vi "LDA1_Safety.vi"(1 "Adam Loop Count":i32, 2 "Ch Names":string[](array[string]), 3 "Values":dbl[](array[numeric]) format="%.2f") -> (0 "Scan comment":string)   [LabVIEW 2014]
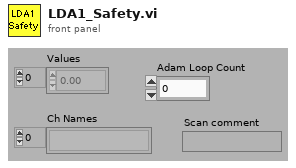
[diagram p1: front panel]
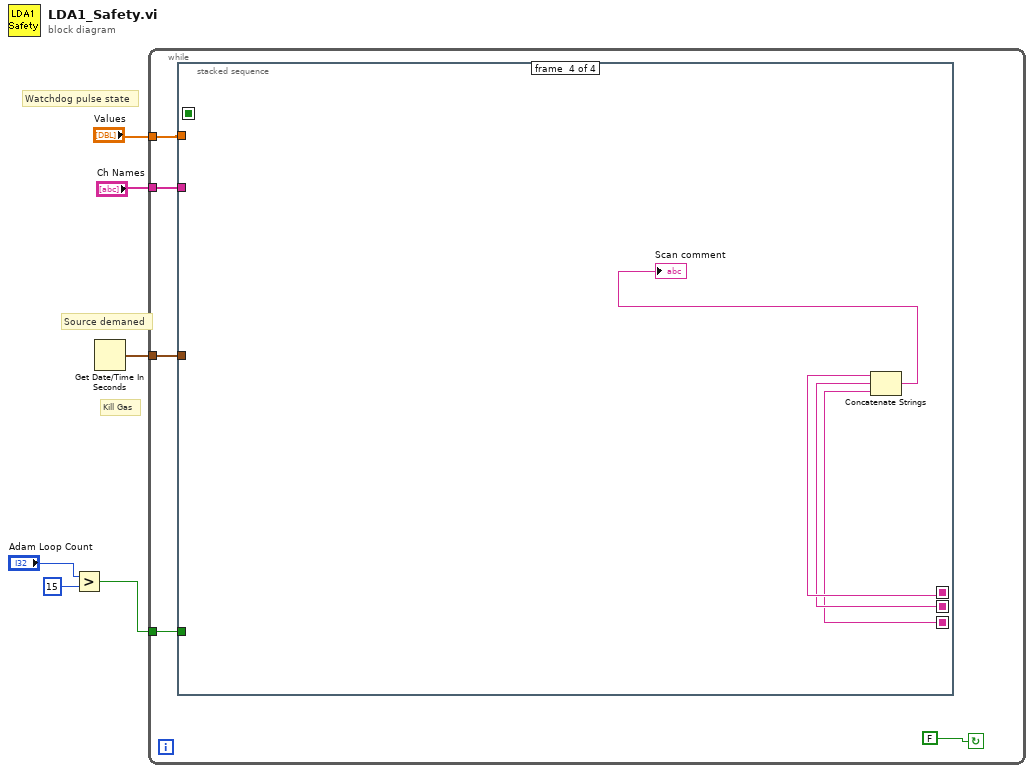
[diagram p0: block diagram]
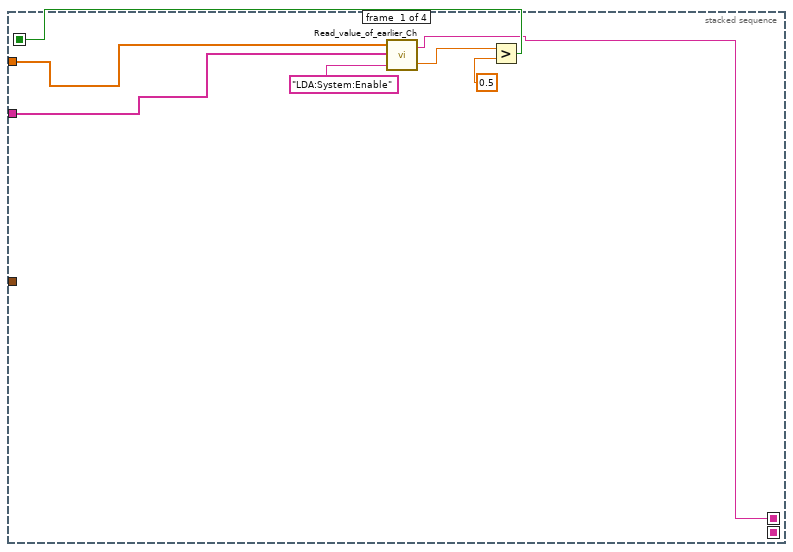
[diagram p2: hidden frame]
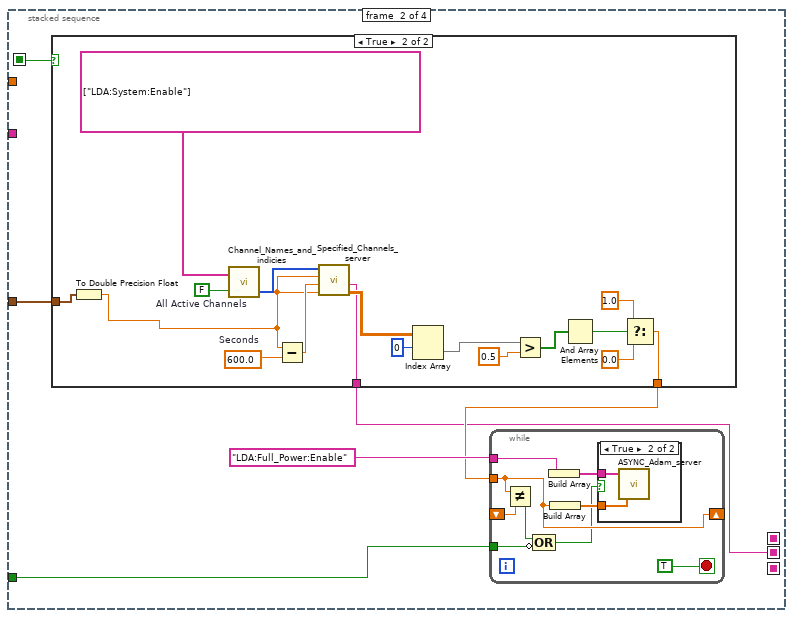
[diagram p3: hidden frame]
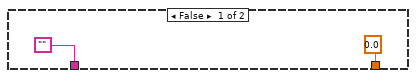
[diagram p5: hidden frame]
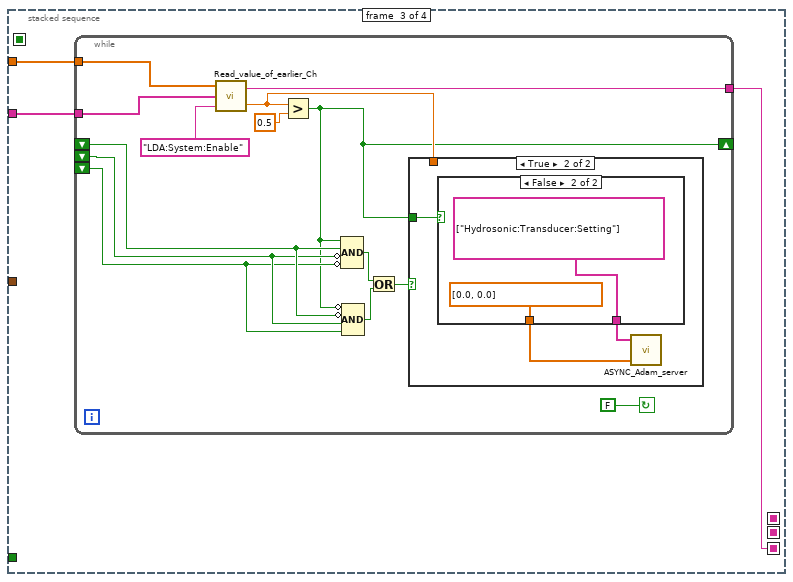
[diagram p6: hidden frame]
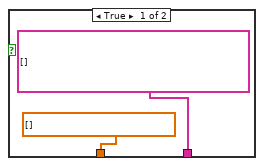
[diagram p8: hidden frame]
diagram:
  # "Source demaned"
  # "Watchdog pulse state"
  # "Kill Gas"
  n1 = Greater?(x="Adam Loop Count", y=15) -> (0:w2:bool)
  n2 = Get Date/Time In Seconds() -> (seconds since 1Jan1904=w1:timestamp)
  n3 = while {
    tunnel: "Ch Names" -> [w11]
    tunnel: "Values" -> [w10]
    tunnel: w2 -> [w8]
    tunnel: w1 -> [w7]
    stop <- FALSE continue-if-true
    n4 = stacked-sequence {
      seq-local: [w16 _ _ _] -> [_ w23 _ _]
      seq-local: [w12 _ _ _] -> [_ _ _ w82]
      seq-local: [_ w19 _ _] -> [_ _ _ w81]
      seq-local: [_ _ w55 _] -> [_ _ _ w80]
      tunnel: w11 -> [w17 _ w56 _]
      tunnel: w10 -> [w18 _ w57 _]
      tunnel: w8 -> [_ w21 _ _]
      tunnel: w7 -> [_ w24 _ _]
      frame #0 {
        n5 = call "Read_value_of_earlier_Ch.vi"("Desired Ch to Read"="LDA:System:Enable", "Ch names"=w17, "Present scan array"=w18) -> ("Value"=w14:dbl, "Scan comment"=w12:string)  [unwired: 1 in]
        n6 = Greater?(x=w14, y=0.5) -> (0:w16:bool)
      }
      frame #1 {
        n7 = case shown="True" w23 {
          tunnel: w24 -> [_ w54]
          tunnel: [0.0 ("y") w42] -> w20
          tunnel: ["" w39] -> w19
          frame False {
          }
          frame True {
            w52 = 600.0  # Seconds
            w50 = FALSE  # All Active Channels
            n8 = To Double Precision Float(number=w54) -> (double precision float=w48:dbl)
            n9 = call "Channel_Names_and_indicies.vi"("All Active Channels"=w50, "Desired Ch Names"=string[] ["LDA:System:Enable"]) -> ("Indicies"=w51:i32[])  [unwired: 1 out]
            n10 = Subtract(x=w48, y=w52) -> (x-y=w53:dbl)
            n11 = call "Specified_Channels_server.vi"("End time"=w48, "Start time"=w53, "Clients time"=w48, "Requested channels"=w51) -> ("Output array"=w46:dbl[][], "Messages"=w39:string)  [unwired: 1 in, 3 out]
            n12 = Index Array(array=w46, index (row)=0) -> (element=w38:dbl[])  [unwired: 1 in]
            n13 = Greater?(x=w38, y=0.5) -> (0:w41:bool[])
            n14 = And Array Elements(Boolean array=w41) -> (logical AND=w40:bool)
            n15 = Select(t=1.0 ("y"), s=w40, f=0.0 ("y")) -> (s? t:f=w42:dbl)
          }
        }
        n16 = while {
          shift-right: [w29] -> _
          shift-left: _ -> [w30]
          tunnel: w20 -> [w29]
          tunnel: "LDA:Full_Power:Enable" -> [w31]
          tunnel: w21 -> [w26]
          stop <- TRUE stop-if-true
          n17 = Not Equal?(x=w29, y=w30) -> (x != y?=w27:bool)
          n18 = Compound Arithmetic op=OR(w27, invert w26) -> (w25:bool)
          n19 = Build Array(w31) -> (w32:string[])
          n20 = Build Array(w29) -> (w33:dbl[])
          n21 = case shown="True" w25 {
            tunnel: w33 -> [_ w35]
            tunnel: w32 -> [_ w34]
            frame False {
            }
            frame True {
              n22 = call "ASYNC_Adam_server.vi"("Values"=w35, "Channel Names"=w34) -> ()  [unwired: 1 in, 3 out]
            }
          }
        }
      }
      frame #2 {
        n23 = while {
          tunnel: w57 -> [w71]
          tunnel: w56 -> [w70]
          shift-right: [w59] -> _
          shift-left: _ -> [w65]
          shift-left: _ -> [w64]
          shift-left: _ -> [w63]
          tunnel: [w58] -> w55
          stop <- FALSE continue-if-true
          n24 = call "Read_value_of_earlier_Ch.vi"("Desired Ch to Read"="LDA:System:Enable", "Ch names"=w70, "Present scan array"=w71) -> ("Value"=w66:dbl, "Scan comment"=w58:string)  [unwired: 1 in]
          n25 = Greater?(x=w66, y=0.5) -> (0:w59:bool)
          n26 = Compound Arithmetic op=AND(w59, w65, invert w64, invert w63) -> (w61:bool)
          n27 = Compound Arithmetic op=AND(invert w59, invert w65, w64, w63) -> (w62:bool)
          n28 = Or(x=w61, y=w62) -> (x .or. y?=w60:bool)
          n29 = case shown="True" w60 {
            tunnel: w66 -> [_ _]
            tunnel: w59 -> [_ w74]
            frame False {
            }
            frame True {
              n30 = case shown="False" w74 {
                tunnel: [string[] [] ("Channel Names") string[] ["Hydrosonic:Transducer:Setting"] ("Channel Names")] -> w73
                tunnel: [dbl[] [] ("Values") dbl[] [0.0, 0.0] ("Values")] -> w72
                frame True {
                }
                frame False {
                }
              }
              n31 = call "ASYNC_Adam_server.vi"("Values"=w72, "Channel Names"=w73) -> ()  [unwired: 1 in, 3 out]
            }
          }
        }
      }
      frame #3 {
        n32 = Concatenate Strings(w82, w81, w80) -> (→"Scan comment":string)
      }
    }
  }
